vi "clear_sts_attributes.vi"   [LabVIEW 2021]
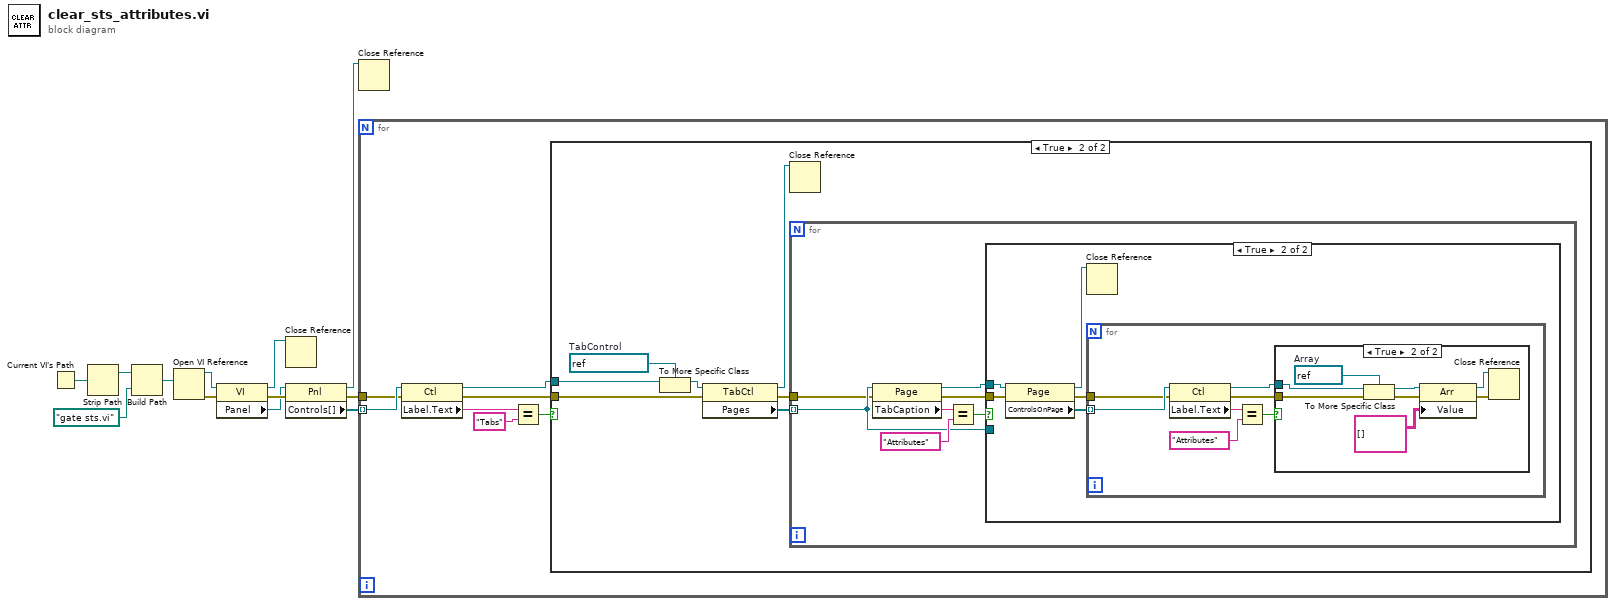
[diagram p0: block diagram]
diagram:
  n1 = Current VI's Path() -> (path=w12:path)
  n2 = Strip Path(path=w12) -> (stripped path=w11:path)  [unwired: 1 out]
  n3 = Build Path(base path=w11, name or relative path=path "gate sts.vi") -> (appended path=w9:path)
  n4 = Open VI Reference(vi path=w9) -> (vi reference=w8:refnum<vi>, error out=w3:errorcluster)  [unwired: 5 in]
  n5 = property class="VI"(reference=w8, error in=w3) -> (reference out=w4:refnum<vi>, error out=w7:errorcluster, "Panel"=w6:refnum<vi>)
  n6 = Close Reference(reference=w4) -> ()  [unwired: 1 in, 1 out]
  n7 = property class="Pnl"(reference=w6, error in=w7) -> (reference out=w2:refnum<vi>, error out=w1:errorcluster, "Controls[]"=w5:refnum<vi>[])
  n8 = Close Reference(reference=w2) -> ()  [unwired: 1 in, 1 out]
  n9 = for {
    tunnel: w5 -> [w19] mode=indexing
    tunnel: w1 -> [w14]
    n10 = property class="Ctl"(reference=w19, error in=w14) -> (reference out=w15:refnum<vi>, error out=w13:errorcluster, "Label.Text"=w18:string)
    n11 = Equal?(x=w18, y="Tabs") -> (x = y?=w16:bool)
    n12 = case shown="True" w16 {
      tunnel: w15 -> [_ w25]
      tunnel: w13 -> [_ w22]
      frame False {
      }
      frame True {
        w26 = refnum<vi> refnum  # TabControl
        n13 = To More Specific Class(target class=w26, reference=w25) -> (specific class reference=w24:refnum<vi>)  [unwired: 1 in, 1 out]
        n14 = property class="TabCtl"(reference=w24, error in=w22) -> (reference out=w20:refnum<vi>, error out=w21:errorcluster, "Pages"=w23:refnum<vi>[])
        n15 = Close Reference(reference=w20) -> ()  [unwired: 1 in, 1 out]
        n16 = for {
          tunnel: w23 -> [w30] mode=indexing
          tunnel: w21 -> [w28]
          n17 = property class="Page"(reference=w30, error in=w28) -> (reference out=w29:refnum<vi>, error out=w27:errorcluster, "TabCaption"=w33:string)
          n18 = Equal?(x=w33, y="Attributes") -> (x = y?=w31:bool)
          n19 = case shown="True" w31 {
            tunnel: w30 -> [_ _]
            tunnel: w29 -> [_ w38]
            tunnel: w27 -> [_ w36]
            frame False {
            }
            frame True {
              n20 = property class="Page"(reference=w38, error in=w36) -> (reference out=w34:refnum<vi>, error out=w35:errorcluster, "ControlsOnPage"=w37:refnum<vi>[])
              n21 = Close Reference(reference=w34) -> ()  [unwired: 1 in, 1 out]
              n22 = for {
                tunnel: w37 -> [w45] mode=indexing
                tunnel: w35 -> [w40]
                n23 = property class="Ctl"(reference=w45, error in=w40) -> (reference out=w41:refnum<vi>, error out=w39:errorcluster, "Label.Text"=w44:string)
                n24 = Equal?(x=w44, y="Attributes") -> (x = y?=w42:bool)
                n25 = case shown="True" w42 {
                  tunnel: w41 -> [_ w53]
                  tunnel: w39 -> [_ w49]
                  frame False {
                  }
                  frame True {
                    w52 = refnum<vi> refnum  # Array
                    n26 = To More Specific Class(target class=w52, reference=w53, error in=w49) -> (specific class reference=w51:refnum<vi>, error out=w48:errorcluster)
                    n27 = property class="Arr"(reference=w51, error in=w48, "Value"=string[][] [] ("Attributes")) -> (reference out=w47:refnum<vi>, error out=w46:errorcluster)
                    n28 = Close Reference(reference=w47, error in (no error)=w46) -> ()  [unwired: 1 out]
                  }
                }
              }
            }
          }
        }
      }
    }
  }
